vi "Vision Processing.vi"(5 "Retroreflective Processing":bool=TRUE, 7 "Team Color Processing":bool=TRUE, 9 "Threshold Values":T1(array[cluster]), 10 "Camera Image":T2(plugin-control)) -> (0 "Particle Reports (Pixels)":T3(array[cluster]) {"Orientation" format="%.2f"; "Dimensions"."Height" format="%.2f"; "Dimensions"."Width" format="%.2f"; "Center of Mass"."Y" format="%.2f"; "Center of Mass"."X" format="%.2f"; "Bounding Rect"."Bottom" format="%.2f"; "Bounding Rect"."Right" format="%.2f"; "Bounding Rect"."Top" format="%.2f"; "Bounding Rect"."Left" format="%.2f"; "Number of Holes" format="%.2f"; "Area" format="%.2f"}, 1 "Number of Particles":i32, 2 "Retro Image":T2(plugin-control), 3 "Annotations":cluster{"Text":string, "X":dbl, "Y":dbl}[](array[cluster]))   [LabVIEW 2013]
uses:
  <vilib>/vision/NI_Vision_Development_Module.lvlib
panel:
  out "Output Image Result":T2(plugin-control)
  out "Blue Image":T2(plugin-control)
  out "Red Image":T2(plugin-control)
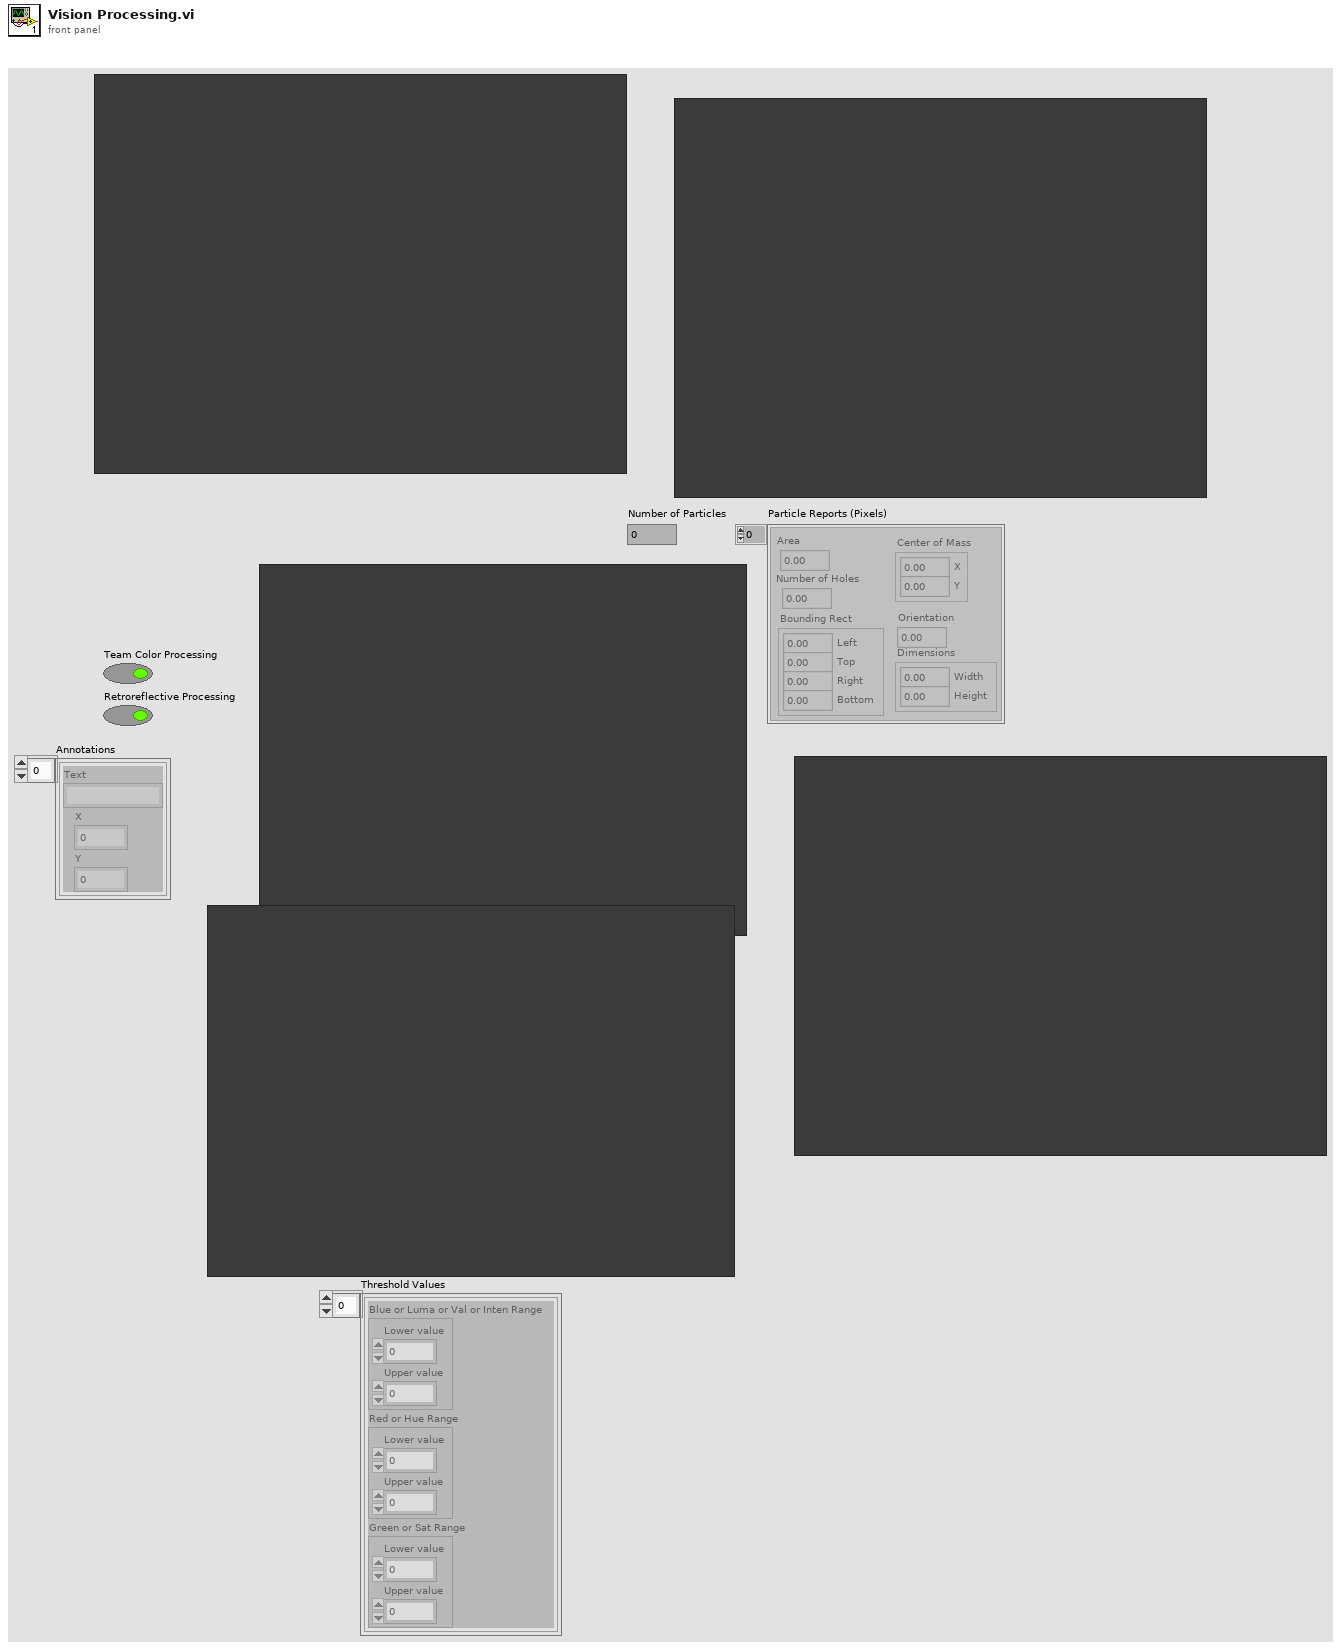
[diagram p1: front panel]
types:
  T1 = cluster{"Blue or Luma or Val or Inten Range":cluster{"Lower value":i32, "Upper value":i32}, "Red or Hue Range":cluster{"Lower value":i32, "Upper value":i32}, "Green or Sat Range":cluster{"Lower value":i32, "Upper value":i32}}[]
  T2 = typedef "IMAQ Image.ctl" = refnum<image>
  T3 = cluster{"Area":dbl, "Number of Holes":dbl, "Bounding Rect":cluster{"Left":dbl, "Top":dbl, "Right":dbl, "Bottom":dbl}, "Center of Mass":cluster{"X":dbl, "Y":dbl}, "Orientation":dbl, "Dimensions":cluster{"Width":dbl, "Height":dbl}}[]
  T4 = cluster{"Threshold Values[0]":cluster{"Blue or Luma or Val or Inten Range":cluster{"Lower value":i32, "Upper value":i32}, "Red or Hue Range":cluster{"Lower value":i32, "Upper value":i32}, "Green or Sat Range":cluster{"Lower value":i32, "Upper value":i32}}, "Threshold Values[1]":cluster{"Blue or Luma or Val or Inten Range":cluster{"Lower value":i32, "Upper value":i32}, "Red or Hue Range":cluster{"Lower value":i32, "Upper value":i32}, "Green or Sat Range":cluster{"Lower value":i32, "Upper value":i32}}, "Threshold Values[2]":cluster{"Blue or Luma or Val or Inten Range":cluster{"Lower value":i32, "Upper value":i32}, "Red or Hue Range":cluster{"Lower value":i32, "Upper value":i32}, "Green or Sat Range":cluster{"Lower value":i32, "Upper value":i32}}, "Threshold Values[3]":cluster{"Blue or Luma or Val or Inten Range":cluster{"Lower value":i32, "Upper value":i32}, "Red or Hue Range":cluster{"Lower value":i32, "Upper value":i32}, "Green or Sat Range":cluster{"Lower value":i32, "Upper value":i32}}, "Threshold Values[4]":cluster{"Blue or Luma or Val or Inten Range":cluster{"Lower value":i32, "Upper value":i32}, "Red or Hue Range":cluster{"Lower value":i32, "Upper value":i32}, "Green or Sat Range":cluster{"Lower value":i32, "Upper value":i32}}, "Threshold Values[5]":cluster{"Blue or Luma or Val or Inten Range":cluster{"Lower value":i32, "Upper value":i32}, "Red or Hue Range":cluster{"Lower value":i32, "Upper value":i32}, "Green or Sat Range":cluster{"Lower value":i32, "Upper value":i32}}, "Threshold Values[6]":cluster{"Blue or Luma or Val or Inten Range":cluster{"Lower value":i32, "Upper value":i32}, "Red or Hue Range":cluster{"Lower value":i32, "Upper value":i32}, "Green or Sat Range":cluster{"Lower value":i32, "Upper value":i32}}, "Threshold Values[7]":cluster{"Blue or Luma or Val or Inten Range":cluster{"Lower value":i32, "Upper value":i32}, "Red or Hue Range":cluster{"Lower value":i32, "Upper value":i32}, "Green or Sat Range":cluster{"Lower value":i32, "Upper value":i32}}, "Threshold Values[8]":cluster{"Blue or Luma or Val or Inten Range":cluster{"Lower value":i32, "Upper value":i32}, "Red or Hue Range":cluster{"Lower value":i32, "Upper value":i32}, "Green or Sat Range":cluster{"Lower value":i32, "Upper value":i32}}}
  T5 = cluster{"Blue or Luma or Val or Inten Range":cluster{"Lower value":i32, "Upper value":i32}, "Red or Hue Range":cluster{"Lower value":i32, "Upper value":i32}, "Green or Sat Range":cluster{"Lower value":i32, "Upper value":i32}}
  T6 = typedef "Particle Parameters" = i32
  T7 = cluster{"Measurement Parameter":T6, "Range Lower Value":dbl, "Range Upper Value":dbl, "Range":bool, "Measurement Type":bool}[]
  T8 = typedef "Image Type" = u32
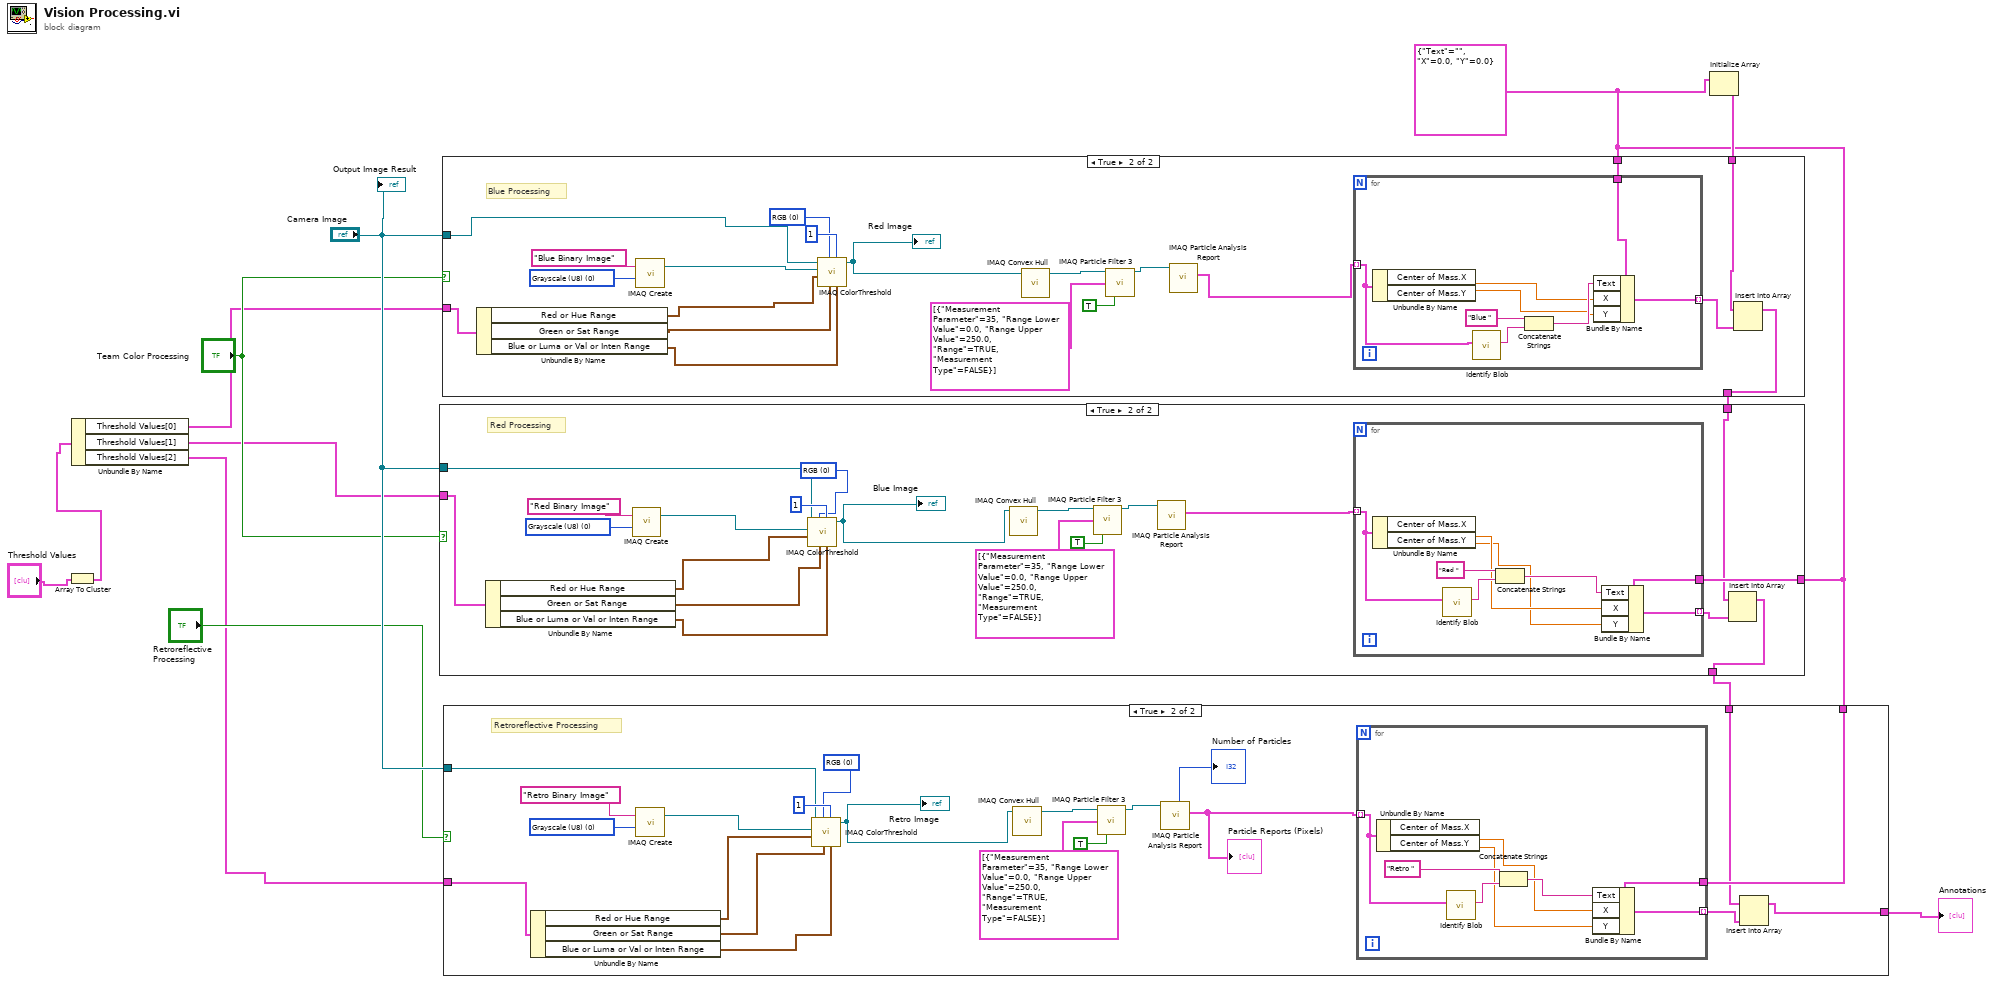
[diagram p0: block diagram]
diagram:
  w8 = cluster{"Text":string, "X":dbl, "Y":dbl} {"Text"="", "X"=0.0, "Y"=0.0}
  n1 = Array To Cluster(array="Threshold Values") -> (cluster=w1:T4)
  n2 = Unbundle By Name(w1) -> ("Threshold Values[0]"=w5:T5, "Threshold Values[1]"=w4:T5, "Threshold Values[2]"=w3:T5)
  n3 = Initialize Array(w8) -> (w10:cluster{"Text":string, "X":dbl, "Y":dbl}[])  [unwired: 1 in]
  n4 = case shown="True" "Team Color Processing" {
    tunnel: "Camera Image" -> [_ w23]
    tunnel: w8 -> [_ w22]
    tunnel: w10 -> [w14 w21]
    tunnel: [w14 w19] -> w9
    tunnel: w5 -> [_ w18]
    frame False {
    }
    frame True {
      w26 = u16 0 items=["RGB", "HSL", "HSV", "HSI"] ("Color Mode")
      w33 = T8 0 items=["Grayscale (U8)", "Grayscale (I16)", "Grayscale (SGL)", "Complex (CSG)", "RGB (U32)", "HSL (U32)", "RGB (U64)", "Grayscale (U16)"] ("Image Type")
      # "Blue Processing"
      n5 = Unbundle By Name(w18) -> ("Red or Hue Range"=w15:cluster{"Lower value":i32, "Upper value":i32}, "Green or Sat Range"=w16:cluster{"Lower value":i32, "Upper value":i32}, "Blue or Luma or Val or Inten Range"=w17:cluster{"Lower value":i32, "Upper value":i32})
      n6 = call "IMAQ Create"("Image Name"="Blue Binary Image", "Image Type"=w33) -> ("New Image"=w32:T2)  [unwired: 3 in, 1 out]
      n7 = call "IMAQ ColorThreshold"("Blue or Luma or Val or Inten Range"=w17, "Replace Value"=1, "Green or Sat Range"=w16, "Color Mode"=w26, "Red or Hue Range"=w15, "Image Dst"=w32, "Image Src"=w23) -> ("Image Dst Out"=w24:T2)  [unwired: 3 in, 1 out]
      "Red Image" <- w24
      n8 = call "IMAQ Convex Hull"("Image Src"=w24) -> ("Image Dst Out"=w30:T2)  [unwired: 9 in, 1 out]
      n9 = call "IMAQ Particle Filter 3"("Image Src"=w30, "Selection Values"=T7 [{"Measurement Parameter"=35, "Range Lower Value"=0.0, "Range Upper Value"=250.0, "Range"=TRUE, "Measurement Type"=FALSE}], "Reject Border? (F)"=TRUE) -> ("Image Dst Out"=w27:T2)  [unwired: 10 in, 2 out]
      n10 = call "IMAQ Particle Analysis Report"("Image"=w27) -> ("Particle Reports (Pixels)"=w25:T3)  [unwired: 5 in, 5 out]
      n11 = for {
        tunnel: w25 -> [w40] mode=indexing
        tunnel: w22 -> [w39]
        tunnel: [w35] -> w20 mode=indexing
        n12 = Unbundle By Name(w40) -> ("Center of Mass.X"=w37:dbl, "Center of Mass.Y"=w36:dbl)
        n13 = call "Identify Blob.vi"("Particle Report"=w40) -> ("Result"=w42:string)  [unwired: 10 in]
        n14 = Concatenate Strings("Blue ", w42) -> (w38:string)
        n15 = Bundle By Name(cluster=w39, "Text"=w38, "X"=w37, "Y"=w36) -> (w35:cluster{"Text":string, "X":dbl, "Y":dbl})
      }
      n16 = Insert Into Array(array=w21, new element=w20) -> (w19:cluster{"Text":string, "X":dbl, "Y":dbl}[])  [unwired: 1 in]
    }
  }
  n17 = case shown="True" "Team Color Processing" {
    tunnel: "Camera Image" -> [_ w52]
    tunnel: w8 -> [_ w51]
    tunnel: w9 -> [w43 w50]
    tunnel: [w43 w48] -> w7
    tunnel: w4 -> [_ w47]
    frame False {
    }
    frame True {
      w53 = u16 0 items=["RGB", "HSL", "HSV", "HSI"] ("Color Mode")
      w63 = T8 0 items=["Grayscale (U8)", "Grayscale (I16)", "Grayscale (SGL)", "Complex (CSG)", "RGB (U32)", "HSL (U32)", "RGB (U64)", "Grayscale (U16)"] ("Image Type")
      # "Red Processing"
      n18 = Unbundle By Name(w47) -> ("Red or Hue Range"=w46:cluster{"Lower value":i32, "Upper value":i32}, "Green or Sat Range"=w45:cluster{"Lower value":i32, "Upper value":i32}, "Blue or Luma or Val or Inten Range"=w44:cluster{"Lower value":i32, "Upper value":i32})
      n19 = call "IMAQ Create"("Image Name"="Red Binary Image", "Image Type"=w63) -> ("New Image"=w60:T2)  [unwired: 3 in, 1 out]
      n20 = call "IMAQ ColorThreshold"("Blue or Luma or Val or Inten Range"=w44, "Replace Value"=1, "Green or Sat Range"=w45, "Color Mode"=w53, "Red or Hue Range"=w46, "Image Dst"=w60, "Image Src"=w52) -> ("Image Dst Out"=w54:T2)  [unwired: 3 in, 1 out]
      "Blue Image" <- w54
      n21 = call "IMAQ Convex Hull"("Image Src"=w54) -> ("Image Dst Out"=w56:T2)  [unwired: 9 in, 1 out]
      n22 = call "IMAQ Particle Filter 3"("Image Src"=w56, "Selection Values"=T7 [{"Measurement Parameter"=35, "Range Lower Value"=0.0, "Range Upper Value"=250.0, "Range"=TRUE, "Measurement Type"=FALSE}], "Reject Border? (F)"=TRUE) -> ("Image Dst Out"=w59:T2)  [unwired: 10 in, 2 out]
      n23 = call "IMAQ Particle Analysis Report"("Image"=w59) -> ("Particle Reports (Pixels)"=w55:T3)  [unwired: 5 in, 5 out]
      n24 = for {
        tunnel: w55 -> [w70] mode=indexing
        tunnel: w51 -> [w65]
        tunnel: [w64] -> w49 mode=indexing
        n25 = Unbundle By Name(w70) -> ("Center of Mass.X"=w67:dbl, "Center of Mass.Y"=w66:dbl)
        n26 = call "Identify Blob.vi"("Particle Report"=w70) -> ("Result"=w69:string)  [unwired: 10 in]
        n27 = Concatenate Strings("Red ", w69) -> (w68:string)
        n28 = Bundle By Name(cluster=w65, "Text"=w68, "X"=w67, "Y"=w66) -> (w64:cluster{"Text":string, "X":dbl, "Y":dbl})
      }
      n29 = Insert Into Array(array=w50, new element=w49) -> (w48:cluster{"Text":string, "X":dbl, "Y":dbl}[])  [unwired: 1 in]
    }
  }
  n30 = case shown="True" "Retroreflective Processing" {
    tunnel: "Camera Image" -> [_ w84]
    tunnel: w8 -> [_ w80]
    tunnel: w7 -> [w72 w79]
    tunnel: [w72 w77] -> w6
    tunnel: w3 -> [_ w76]
    frame False {
    }
    frame True {
      w81 = u16 0 items=["RGB", "HSL", "HSV", "HSI"] ("Color Mode")
      w93 = T8 0 items=["Grayscale (U8)", "Grayscale (I16)", "Grayscale (SGL)", "Complex (CSG)", "RGB (U32)", "HSL (U32)", "RGB (U64)", "Grayscale (U16)"] ("Image Type")
      # "Retroreflective Processing"
      n31 = Unbundle By Name(w76) -> ("Red or Hue Range"=w75:cluster{"Lower value":i32, "Upper value":i32}, "Green or Sat Range"=w74:cluster{"Lower value":i32, "Upper value":i32}, "Blue or Luma or Val or Inten Range"=w73:cluster{"Lower value":i32, "Upper value":i32})
      n32 = call "IMAQ Create"("Image Name"="Retro Binary Image", "Image Type"=w93) -> ("New Image"=w90:T2)  [unwired: 3 in, 1 out]
      n33 = call "IMAQ ColorThreshold"("Blue or Luma or Val or Inten Range"=w73, "Replace Value"=1, "Green or Sat Range"=w74, "Color Mode"=w81, "Red or Hue Range"=w75, "Image Dst"=w90, "Image Src"=w84) -> ("Image Dst Out"=w85:T2)  [unwired: 3 in, 1 out]
      "Retro Image" <- w85
      n34 = call "IMAQ Convex Hull"("Image Src"=w85) -> ("Image Dst Out"=w86:T2)  [unwired: 9 in, 1 out]
      n35 = call "IMAQ Particle Filter 3"("Image Src"=w86, "Selection Values"=T7 [{"Measurement Parameter"=35, "Range Lower Value"=0.0, "Range Upper Value"=250.0, "Range"=TRUE, "Measurement Type"=FALSE}], "Reject Border? (F)"=TRUE) -> ("Image Dst Out"=w89:T2)  [unwired: 10 in, 2 out]
      n36 = call "IMAQ Particle Analysis Report"("Image"=w89) -> ("Particle Reports (Pixels)"=w82:T3, "Number of Particles"=→"Number of Particles":i32)  [unwired: 5 in, 4 out]
      "Particle Reports (Pixels)" <- w82
      n37 = for {
        tunnel: w82 -> [w100] mode=indexing
        tunnel: [w95] -> w78 mode=indexing
        tunnel: w80 -> [w94]
        n38 = Unbundle By Name(w100) -> ("Center of Mass.X"=w96:dbl, "Center of Mass.Y"=w97:dbl)
        n39 = call "Identify Blob.vi"("Particle Report"=w100) -> ("Result"=w99:string)  [unwired: 10 in]
        n40 = Concatenate Strings("Retro ", w99) -> (w98:string)
        n41 = Bundle By Name(cluster=w94, "Text"=w98, "X"=w96, "Y"=w97) -> (w95:cluster{"Text":string, "X":dbl, "Y":dbl})
      }
      n42 = Insert Into Array(array=w79, new element=w78) -> (w77:cluster{"Text":string, "X":dbl, "Y":dbl}[])  [unwired: 1 in]
    }
  }
  "Annotations" <- w6
  "Output Image Result" <- "Camera Image"
